vi "Set XY Acceleration.vi"(8 "error in (no error)":errorcluster, 10 "mm/s":dbl=200.0 format="%#_13g", 11 "Gantry In":refnum<k24>) -> (0 "error out":errorcluster, 2 "Array":dbl[](array[numeric]), 3 "Gantry Out":refnum<k24>)   [LabVIEW 2020, in "A3200.lvclass"]
uses:
  A3200.lvclass
  Drivers/Aerotech A3200/Aerotech.lvlib
  C:/Program Files (x86)/Aerotech/A3200/LabVIEW/2010/Bin/Aerotech.A3200.dll
  Program Files (x86)/Aerotech/A3200/LabVIEW/2010/Bin/Aerotech.A3200.dll
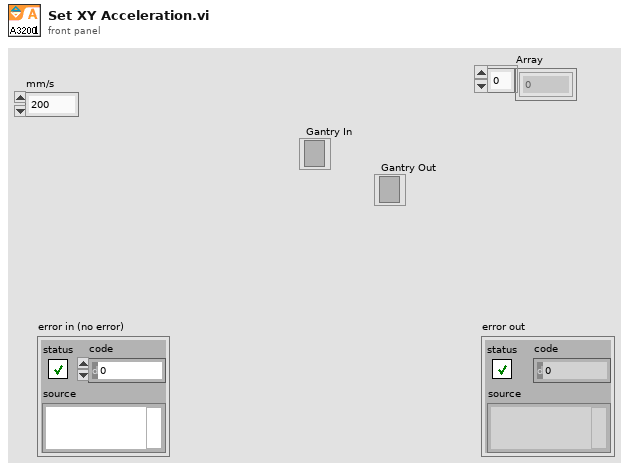
[diagram p1: front panel]
types:
  T1 = cluster{"Status":bool, "Error Code":i32, "Source":string}
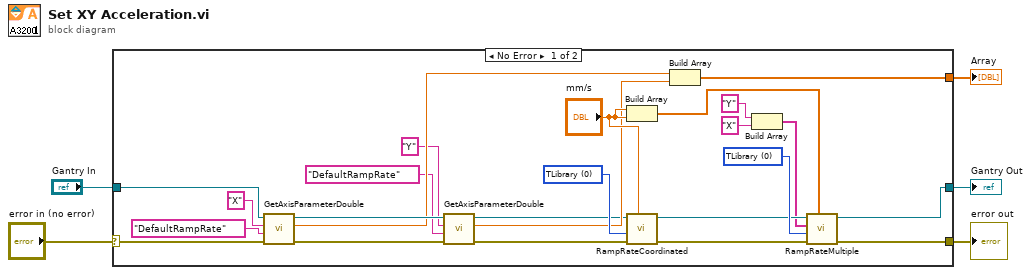
[diagram p0: block diagram]
diagram:
  n1 = case shown="No Error" "error in (no error)" {
    selector: "error in (no error)" -> [w6 w31]
    tunnel: [w29 _] -> w5
    tunnel: [w28 w31] -> w4
    tunnel: "Gantry In" -> [w27 w30]
    tunnel: [w26 w30] -> w2
    frame No Error {
      w23 = 0 items=["TLibrary", "T01", "T02", "T03", "T04", "T05", "T06", "T07", "T08", "T09", "T10", "T11", "T12", "T13", "T14", "T15", "T16", "T17", "T18", "T19", "T20", "T21", "T22", "T23", "T24", "T25", "T26", "T27", "T28", "T29", "T30", "T31"] ("task id")
      w24 = 0 items=["TLibrary", "T01", "T02", "T03", "T04", "T05", "T06", "T07", "T08", "T09", "T10", "T11", "T12", "T13", "T14", "T15", "T16", "T17", "T18", "T19", "T20", "T21", "T22", "T23", "T24", "T25", "T26", "T27", "T28", "T29", "T30", "T31"] ("taskId")
      n2 = call "GetAxisParameterDouble.vi"("error in (no error)"=w6, "Parameter Name"="DefaultRampRate", "axis name"="X", "controller in"=w27) -> ("error out"=w12:errorcluster, "value"=w13:dbl, "controller out"=w14:refnum<k24>)  [unwired: 5 in]
      n3 = call "GetAxisParameterDouble.vi"("error in (no error)"=w12, "Parameter Name"="DefaultRampRate", "axis name"="Y", "controller in"=w14) -> ("error out"=w11:errorcluster, "value"=w10:dbl, "controller out"=w9:refnum<k24>)  [unwired: 5 in]
      n4 = Build Array("mm/s", "mm/s") -> (w25:dbl[])
      n5 = call "RampRateCoordinated.vi"("ramp rate"="mm/s", "error in (no error)"=w11, "taskId"=w24, "controller in"=w9) -> ("error out"=w17:T1, "controller out"=w22:refnum<k24>)  [unwired: 6 in]
      n6 = Build Array(w13, w10) -> (w29:dbl[])
      n7 = Build Array("Y", "X") -> (w19:string[])
      n8 = call "RampRateMultiple.vi"("ramp rates"=w25, "error in (no error)"=w17, "task id"=w23, "axis names"=w19, "controller in"=w22) -> ("error out (no error)"=w28:T1, "controller out"=w26:refnum<k24>)  [unwired: 5 in]
    }
    frame Error {
    }
  }
  "error out" <- w4
  "Array" <- w5
  "Gantry Out" <- w2
